vi "(TestVI)Release Server Test.vi"   [LabVIEW 2020]
uses:
  <vilib>/httpClient/LabVIEWHTTPClient.lvlib
  <vilib>/zip/NI_Unzip.lvlib
types:
  T1 = typedef "LabVIEWHTTPClient.lvlib/ClientHandle.ctl" = refnum<k1>
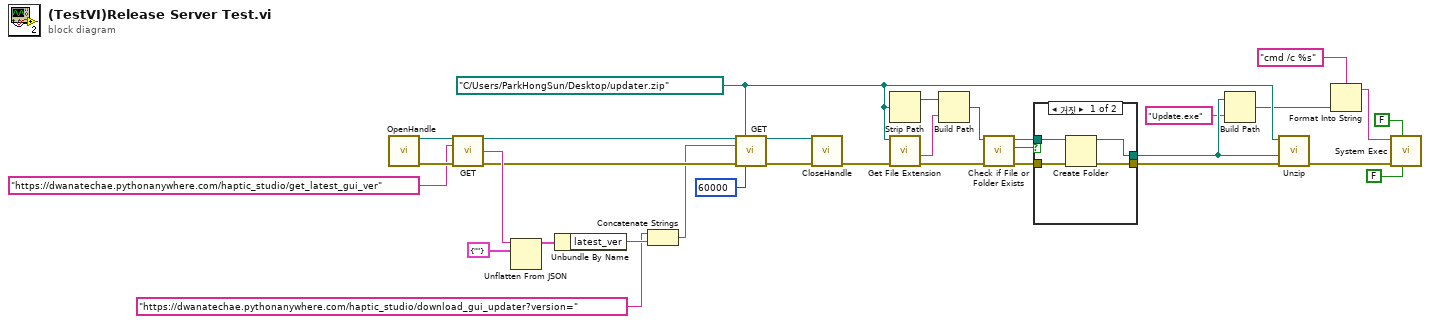
[diagram p0: block diagram]
diagram:
  w18 = path "C:/Users/ParkHongSun/Desktop/updater.zip" ("output file")
  n1 = call <vilib>:"OpenHandle.vi"() -> ("client handle out"=w32:T1, "error out"=w31:errorcluster)  [unwired: 14 in]
  n2 = call <vilib>:"GET.vi"("client handle"=w32, "url"="https://dwanatechae.pythonanywhere.com/haptic_studio/get_latest_gui_ver", "error in (no error)"=w31) -> ("client handle out"=w26:T1, "body"=w29:string, "error out"=w25:errorcluster)  [unwired: 9 in, 1 out]
  n3 = Unflatten From JSON(JSON string=w29, type and defaults=cluster{"latest_ver":string} {"latest_ver"=""}) -> (value=w27:cluster{"latest_ver":string})  [unwired: 5 in, 1 out]
  n4 = Unbundle By Name(w27) -> ("latest_ver"=w22:string)
  n5 = Concatenate Strings("https://dwanatechae.pythonanywhere.com/haptic_studio/download_gui_updater?version=" ("url"), w22) -> (w20:string)
  n6 = call <vilib>:"GET.vi"("client handle"=w26, "output file"=w18, "url"=w20, "error in (no error)"=w25, "timeout (10000)"=60000) -> ("client handle out"=w24:T1, "error out"=w23:errorcluster)  [unwired: 7 in, 2 out]
  n7 = call <vilib>:"CloseHandle.vi"("client handle"=w24, "error in (no error)"=w23) -> ("error out"=w19:errorcluster)  [unwired: 13 in]
  n8 = Strip Path(path=w18) -> (stripped path=w17:path)  [unwired: 1 out]
  n9 = call <vilib>:"Get File Extension.vi"("error in (no error)"=w19, "file"=w18) -> ("error out"=w15:errorcluster, "filename without extension"=w16:string)  [unwired: 5 in, 3 out]
  n10 = Build Path(base path=w17, name or relative path=w16) -> (appended path=w14:path)
  n11 = call <vilib>:"Check if File or Folder Exists.vi"("error in (no error)"=w15, "path"=w14) -> ("error out"=w13:errorcluster, "file or folder exists?"=w11:bool, "dup path"=w12:path)  [unwired: 7 in]
  n12 = case shown="거짓" w11 {
    tunnel: w13 -> [w36 w37]
    tunnel: w12 -> [w35 w38]
    tunnel: [w34 w38] -> w9
    tunnel: [w33 w37] -> w10
    frame False {
      n13 = Create Folder(path (use dialog)=w35, error in=w36) -> (created path=w34:path, error out=w33:errorcluster)  [unwired: 1 in, 1 out]
    }
    frame True {
    }
  }
  n14 = Build Path(base path=w9, name or relative path="Update.exe" ("이름 또는 상대 경로")) -> (appended path=w5:path)
  n15 = call <vilib>:"Unzip.vi"("error in (no error)"=w10, "Target directory (same as Zip file if empty)"=w9, "Zip file"=w18) -> ("error out"=w7:errorcluster)  [unwired: 6 in, 2 out]
  n16 = Format Into String(format string="cmd /c %s" ("포맷 문자열"), w5) -> (resulting string=w4:string)  [unwired: 2 in, 1 out]
  n17 = call <vilib>:"System Exec.vi"("run minimized? (F)"=FALSE, "wait until completion? (T)"=FALSE, "error in (no error)"=w7, "command line"=w4) -> ()  [unwired: 4 in, 4 out]
